vi "filter.vi"(8 "error in":errorcluster, 11 "data_in":T1 {"config"."updateTime" format="%#_g ms"; "config"."lowPass" format="%#_g Hz"; "config"."highPass" format="%#_g Hz"; "config"."cutoff" format="%#_g dB"; "config"."preTrigger" format="%#_g ms"; "config"."thr" format="%#_g N"; "config"."duration" format="%#_g s"; "config"."rate" min=1652.0 max=51200.0 format="%#_g Hz"}) -> (0 "error out":errorcluster, 3 "data_out":T1 {"config"."updateTime" format="%#_g ms"; "config"."lowPass" format="%#_g Hz"; "config"."highPass" format="%#_g Hz"; "config"."cutoff" format="%#_g dB"; "config"."preTrigger" format="%#_g ms"; "config"."thr" format="%#_g N"; "config"."duration" format="%#_g s"; "config"."rate" min=1652.0 max=51200.0 format="%#_g Hz"})   [LabVIEW 2016]
uses:
  results_data.ctl
  MainFGV/Settings/Advanced/AdvancedConfig.ctl
  <vilib>/Analysis/3filter.llb/Filter Passband Type.ctl
  <vilib>/Analysis/baseanly.llb/Mean (DBL).vi
  <vilib>/Analysis/3filter.llb/Butterworth Filter (DBL).vi
  <vilib>/Analysis/NI_AALBase.lvlib
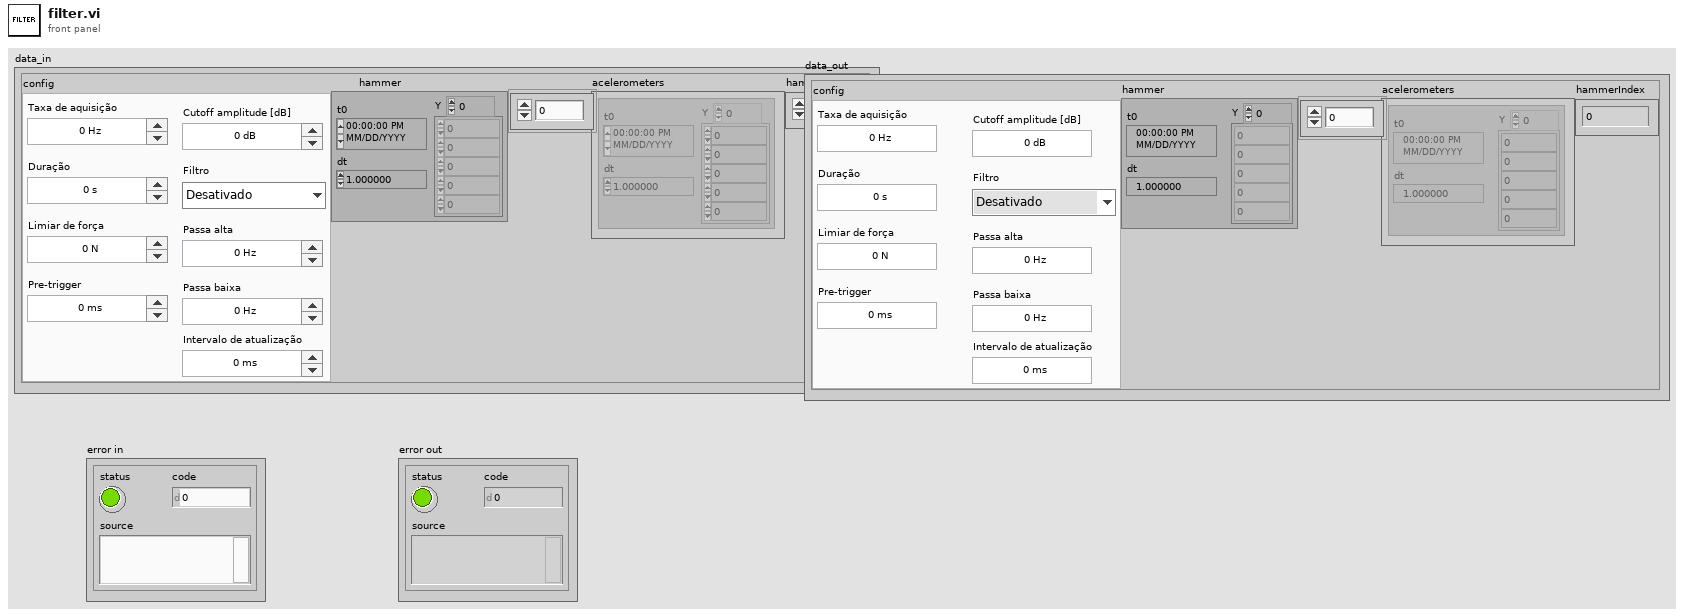
[diagram p1: front panel]
types:
  T1 = typedef "results_data.ctl" = cluster{"config":T2, "hammer":waveform(dbl), "acelerometers":waveform(dbl)[], "hammerIndex":i32}
  T2 = typedef "AdvancedConfig.ctl" = cluster{"rate":dbl, "duration":dbl, "thr":dbl, "preTrigger":dbl, "cutoff":dbl, "Filtro":enum16{"Desativado", "Passa banda", "Passa alta", "Passa baixa"}, "highPass":dbl, "lowPass":dbl, "updateTime":dbl}
  T3 = enum16{"Desativado", "Passa banda", "Passa alta", "Passa baixa"}
  T4 = typedef "NI_AALBase.lvlib/Filter Passband Type.ctl" = enum32{"Lowpass", "Highpass", "Bandpass", "Bandstop"}
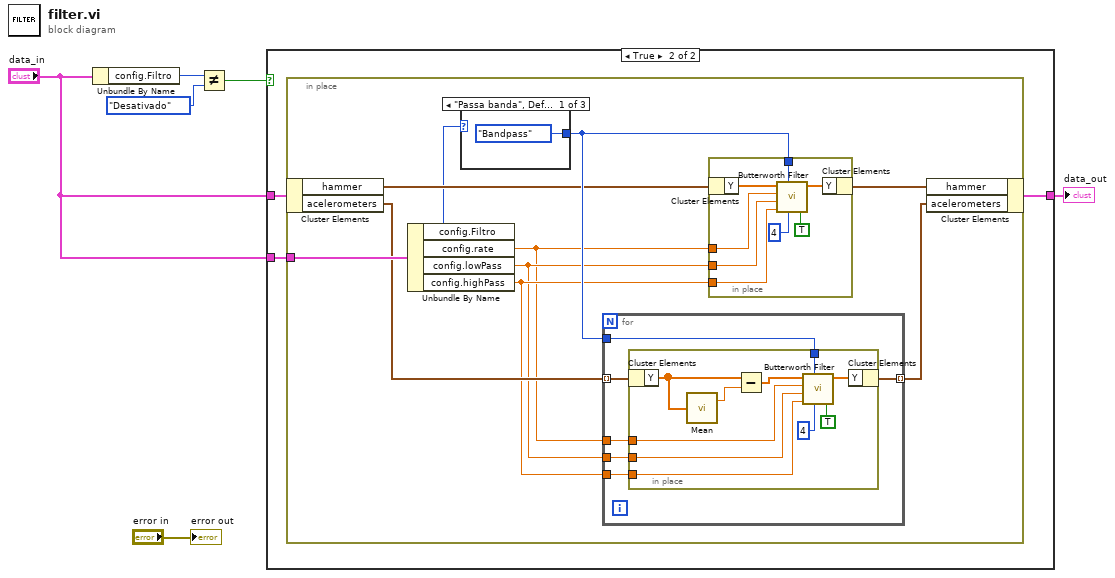
[diagram p0: block diagram]
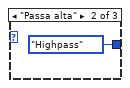
[diagram p3: hidden frame]
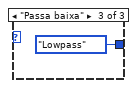
[diagram p4: hidden frame]
diagram:
  n1 = Unbundle By Name("data_in") -> ("config.Filtro"=w6:T3)
  n2 = Not Equal?(x=w6, y=T3."Desativado") -> (x != y?=w4:bool)
  n3 = case shown="True" w4 {
    tunnel: "data_in" -> [w7 w10]
    tunnel: [w7 w8] -> w3
    tunnel: "data_in" -> [_ w9]
    frame False {
    }
    frame True {
      n4 = in-place {
        in-place-border: w9 -> [w18]
        n5 = in-place-cluster #1(w10) -> ("hammer"=w19:waveform(dbl), "acelerometers"=w16:waveform(dbl)[])
        n6 = Unbundle By Name(w18) -> ("config.Filtro"=w15:T3, "config.rate"=w12:dbl, "config.lowPass"=w13:dbl, "config.highPass"=w14:dbl)
        n7 = case shown="\"Passa banda\", Default" w15 {
          tunnel: [Filter_Passband_Type."Bandpass" ("filter type") Filter_Passband_Type."Highpass" ("filter type") Filter_Passband_Type."Lowpass" ("filter type")] -> w20
          frame "Passa banda", Default {
          }
          frame "Passa alta" {
          }
          frame "Passa baixa" {
          }
        }
        n8 = for {
          tunnel: w16 -> [w26] mode=indexing
          tunnel: w14 -> [w25]
          tunnel: w13 -> [w24]
          tunnel: w12 -> [w23]
          tunnel: w20 -> [w22]
          tunnel: [w21] -> w11 mode=indexing
          n9 = in-place {
            in-place-border: w23 -> [w34]
            in-place-border: w24 -> [w33]
            in-place-border: w25 -> [w32]
            in-place-border: w22 -> [w31]
            n10 = in-place-cluster #2(w26) -> ("Y"=w29:dbl[])
            n11 = call-poly <vilib>:"Mean.vi"("X"=w29) -> ("mean"=w28:dbl)  [unwired: 1 out]
            n12 = Subtract(x=w29, y=w28) -> (x-y=w27:dbl[])
            n13 = call-poly <vilib>:"Butterworth Filter.vi"("init/cont (init:F)"=TRUE, "order"=4, "filter type"=w31, "low cutoff freq: fl"=w32, "high cutoff freq: fh"=w33, "sampling freq: fs"=w34, "X"=w27) -> ("Filtered X"=w35:dbl[])  [unwired: 1 in, 1 out]
            n14 = in-place-cluster #2("Y"=w35) -> (w21:waveform(dbl))
          }
        }
        n15 = in-place {
          in-place-border: w20 -> [w44]
          in-place-border: w12 -> [w43]
          in-place-border: w13 -> [w42]
          in-place-border: w14 -> [w41]
          n16 = in-place-cluster #3(w19) -> ("Y"=w46:dbl[])
          n17 = call-poly <vilib>:"Butterworth Filter.vi"("init/cont (init:F)"=TRUE, "order"=4, "filter type"=w44, "low cutoff freq: fl"=w41, "high cutoff freq: fh"=w42, "sampling freq: fs"=w43, "X"=w46) -> ("Filtered X"=w45:dbl[])  [unwired: 1 in, 1 out]
          n18 = in-place-cluster #3("Y"=w45) -> (w17:waveform(dbl))
        }
        n19 = in-place-cluster #1("hammer"=w17, "acelerometers"=w11) -> (w8:T1)
      }
    }
  }
  "data_out" <- w3
  "error out" <- "error in"
